vi "Restore.vi"(8 "error in (no error)":errorcluster, 9 "Previous Version":T1, 10 "Data":string, 11 "Persistent Path Selector in":refnum<class "MGI Persistent Path Selector.lvclass">) -> (0 "error out":errorcluster, 3 "Persistent Path Selector in":refnum<class "MGI Persistent Path Selector.lvclass">)   [LabVIEW 2020, in "MGI Persistent Path Selector.lvclass"]
uses:
  <userlib>/_MGI/User Interface/Path Selector XControl/Class Hierarchy/Persistent Path Selector/MGI Persistent Path Selector.lvclass
  <vilib>/_xctls/Version.ctl
  <userlib>/_MGI/User Interface/Path Selector XControl/Class Hierarchy/Persistent Path Selector/MGI Persistent Path Selector.lvclass/MGI Persistent Path Selector.ctl
  <userlib>/_OpenG.lib/file/file.llb/Valid Path - Traditional__ogtk.vi
  <userlib>/_MGI/User Interface/Path Selector XControl/Class Hierarchy/MGI Path Selector.lvclass
  <vilib>/Utility/VariantDataType/VariantType.lvlib
  <vilib>/_xctls/XControlSupport.lvlib
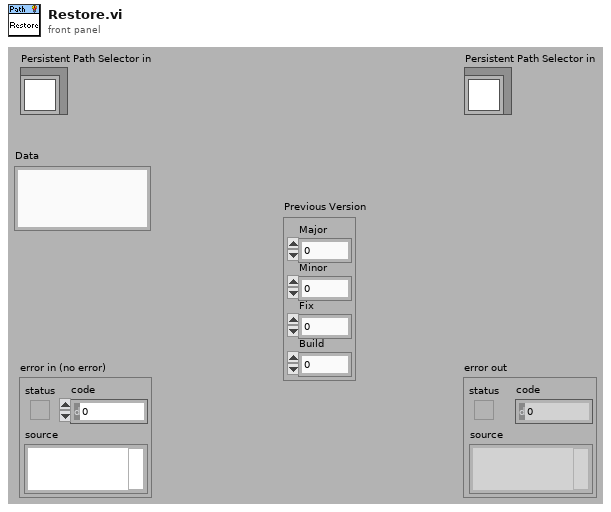
[diagram p1: front panel]
types:
  T1 = typedef "XControlSupport.lvlib/Version.ctl" = cluster{"Major":u16, "Minor":u16, "Fix":u16, "Build":u16}
  T2 = typedef "MGI Persistent Path Selector.lvclass/Persistent Data Cluster.ctl" = cluster{"Initial Path":path, "INI Path":path, "INI Section":string, "Select Option?":bool, "Explorer Option?":bool, "Recurse?":bool, "Allow New?":bool, "Filter":string}
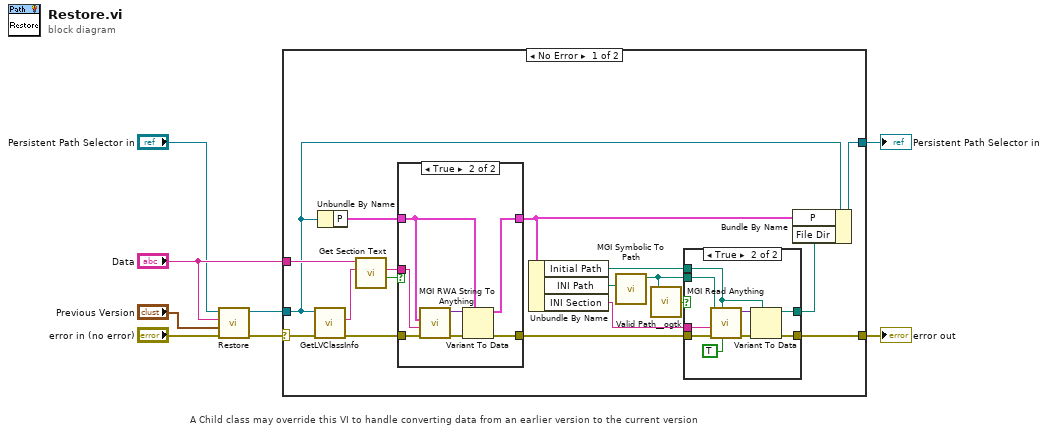
[diagram p0: block diagram]
diagram:
  # "A Child class may override this VI to handle converting data from an earlier version to the current version"
  n1 = call-parent "Restore.vi"("error in (no error)"="error in (no error)", "Previous Version"="Previous Version", "Data"="Data", "Path Selector in"="Persistent Path Selector in") -> ("error out"=w3:errorcluster, "Path Selector out"=w1:refnum<class "MGI Persistent Path Selector.lvclass">)  [unwired: 6 in]
  n2 = case shown="No Error" w3 {
    selector: w3 -> [w13 w48]
    tunnel: [w15 w48] -> w8
    tunnel: [w21 w47] -> w7
    tunnel: w1 -> [w12 w47]
    tunnel: "Data" -> [w22 _]
    frame No Error {
      n3 = call <vilib>:"GetLVClassInfo.vi"("error in (no error)"=w13, "Variant"=w12) -> ("error out"=w26:errorcluster, "LV Class File Name"=w25:string)  [unwired: 7 in, 1 out]
      n4 = Unbundle By Name(w12) -> ("P"=w20:T2)
      n5 = call <userlib>:"Get Section Text.vi"("Section Name"=w25, "Data"=w22) -> ("Section Found?"=w23:bool, "Section Text"=w24:string)  [unwired: 8 in]
      n6 = case shown="True" w23 {
        tunnel: w26 -> [w39 w44]
        tunnel: [w39 w43] -> w14
        tunnel: w24 -> [_ w42]
        tunnel: w20 -> [w38 w41]
        tunnel: [w38 w40] -> w19
        frame False {
        }
        frame True {
          n7 = call <userlib>:"MGI RWA String To Anything.vi"("Error In"=w44, "String"=w42, "Type of Anything"=w41) -> ("Error Out"=w45:errorcluster, "Variant"=w46:variant)  [unwired: 6 in, 1 out]
          n8 = Variant To Data(error in=w45, type=w41, Variant=w46) -> (data=w40:T2, error out=w43:errorcluster)
        }
      }
      n9 = Unbundle By Name(w19) -> ("Initial Path"=w18:path, "INI Path"=w10:path, "INI Section"=w16:string)
      n10 = call <userlib>:"MGI Symbolic To Path.vi"("Symbolic Path"=w10) -> ("Path"=w9:path)  [unwired: 8 in, 2 out]
      n11 = call-poly <userlib>:"Valid Path__ogtk.vi"("path"=w9) -> ("valid"=w11:bool)
      n12 = case shown="True" w11 {
        tunnel: w18 -> [w27 w35]
        tunnel: [w27 w34] -> w17
        tunnel: w16 -> [_ w33]
        tunnel: [w28 w32] -> w15
        tunnel: w14 -> [w28 w31]
        tunnel: w9 -> [_ w29]
        frame False {
        }
        frame True {
          n13 = call <userlib>:"MGI Read Anything.vi"("Use Supplied (F: Use Default)"=TRUE, "Type of Anything"=w35, "Error In"=w31, "Section Name (Name of \"Type of Anything\")"=w33, "Path (dialog)"=w29) -> ("Error Out"=w37:errorcluster, "Anything"=w36:variant)  [unwired: 3 in, 2 out]
          n14 = Variant To Data(error in=w37, type=w35, Variant=w36) -> (data=w34:path, error out=w32:errorcluster)
        }
      }
      n15 = Bundle By Name(cluster=w12, "P"=w19, "File Dir"=w17) -> (w21:refnum<class "MGI Persistent Path Selector.lvclass">)
    }
    frame Error {
    }
  }
  "error out" <- w8
  "Persistent Path Selector in" <- w7
